vi "RFID Get ID Test-2.vi"() -> ()   [LabVIEW 2018]
uses:
  <vilib>/Instr/_visa.llb/VISA Configure Serial Port (Instr).vi
panel:
  out "error out":errorcluster
  in  "Cancel Button":bool
  in  "Get RFID":bool
  out "received":string
  in  "ComPort":refnum<visa-resource-name>="COM10"
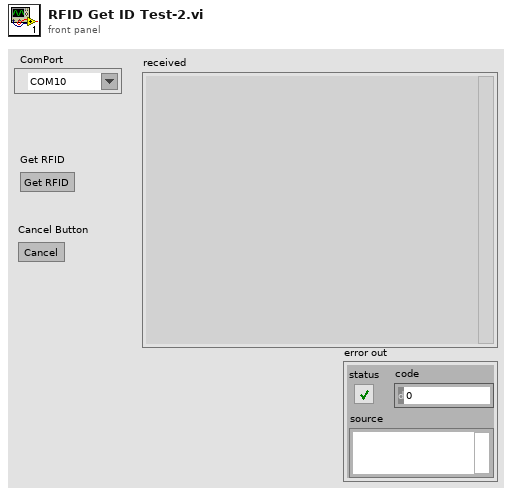
[diagram p1: front panel]
types:
  T1 = enum8{"Enabled", "Disabled", "Disabled and Grayed Out"}
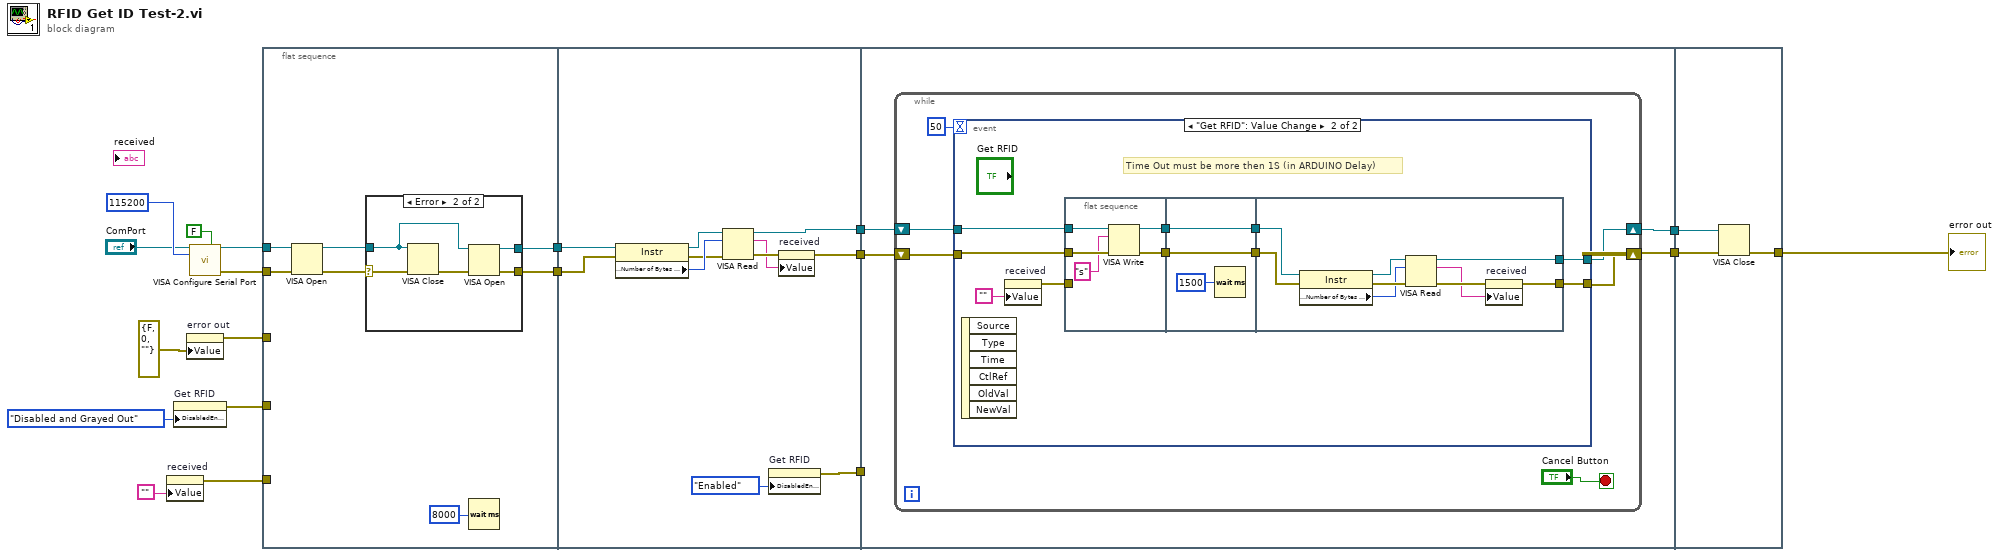
[diagram p0: block diagram]
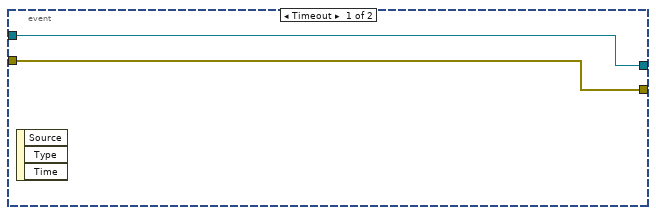
[diagram p3: hidden frame]
diagram:
  n1 = property on="received" class="Str"("Value"="") -> (error out=w13:errorcluster)  [unwired: 2 in, 1 out]
  n2 = property on="Get RFID" class="Bool"("DisabledEnum"=T1."Disabled and Grayed Out" ("Disabled")) -> (error out=w7:errorcluster)  [unwired: 2 in, 1 out]
  n3 = property on="error out" class="Clust (strict)"("Value"=errorcluster {"status"=FALSE, "code"=0, "source"=""} ("error out")) -> (error out=w1:errorcluster)  [unwired: 2 in, 1 out]
  n4 = call-poly "VISA Configure Serial Port"("VISA resource name"="ComPort", "Enable Termination\nChar (T)"=FALSE ("Enable Termination\nChar (T)"), "baud rate (9600)"=u32 115200 ("Serial Settings:Baud Rate")) -> ("VISA resource name out"=w15:refnum<visa-resource-name>, "error out"=w16:errorcluster)  [unwired: 11 in]
  n5 = flat-sequence {
    tunnel: w16 -> [w25]
    tunnel: w15 -> [w24]
    tunnel: w13 -> [_]
    tunnel: w7 -> [_]
    tunnel: [w21] -> w5
    tunnel: [w20] -> w3
    tunnel: w1 -> [_]
    tunnel: [w41] -> w14
    tunnel: [w35] -> w11
    tunnel: [w40] -> w6
    tunnel: w5 -> [w38]
    tunnel: w3 -> [w37]
    tunnel: w14 -> [w48]
    tunnel: w11 -> [w47]
    tunnel: [w46] -> w10
    tunnel: [w45] -> w9
    tunnel: w6 -> [_]
    tunnel: w10 -> [w86]
    tunnel: w9 -> [w85]
    tunnel: [w84] -> w4
    frame #0 {
      n6 = VISA Open(error in (no error)=w25, VISA resource name=w24) -> (VISA resource name=w22:refnum<visa-resource-name>, error out=w23:errorcluster)  [unwired: 3 in]
      n7 = case shown="Error" w23 {
        selector: w23 -> [w27 w33]
        tunnel: w22 -> [w28 w31]
        tunnel: [w28 w30] -> w21
        tunnel: [w27 w29] -> w20
        frame No Error {
        }
        frame Error {
          n8 = VISA Close(VISA resource name=w31, error in (no error)=w33) -> (error out=w32:errorcluster)
          n9 = VISA Open(error in (no error)=w32, VISA resource name=w31) -> (VISA resource name=w30:refnum<visa-resource-name>, error out=w29:errorcluster)  [unwired: 3 in]
        }
      }
      n10 = Wait (ms)(milliseconds to wait=u32 8000) -> ()  [unwired: 1 out]
    }
    frame #1 {
      n11 = property class="Instr"(reference=w38, error in=w37) -> (reference out=w43:refnum<visa-resource-name>, error out=w42:errorcluster, "Serial Settings:Number of Bytes at Serial Port"=w44:u32)
      n12 = VISA Read(VISA resource name=w43, byte count=w44, error in (no error)=w42) -> (VISA resource name out=w41:refnum<visa-resource-name>, read buffer=w34:string, error out=w36:errorcluster)  [unwired: 1 out]
      n13 = property on="Get RFID" class="Bool"("DisabledEnum"=T1."Enabled" ("Disabled")) -> (error out=w40:errorcluster)  [unwired: 2 in, 1 out]
      n14 = property on="received" class="Str"(error in=w36, "Value"=w34) -> (error out=w35:errorcluster)  [unwired: 1 in, 1 out]
    }
    frame #2 {
      n15 = while {
        shift-right: [w52] -> w46
        shift-left: w48 -> [w54]
        shift-right: [w51] -> w45
        shift-left: w47 -> [w53]
        stop <- "Cancel Button" stop-if-true
        n16 = event shown="[1] \"Get RFID\": Value Change" {
          selector: _ -> [_ _]
          dyn-events: _ -> [_ _]
          timeout: 50 -> [_ _]
          tunnel: w54 -> [w56 w66]
          tunnel: w53 -> [w55 w65]
          tunnel: [w56 w60] -> w52
          tunnel: [w55 w59] -> w51
          event Timeout {
            n17 = event-data() -> ()  [unwired: 1 in, 3 out]
          }
          event "Get RFID": Value Change {
            # "Time Out must be more then 1S (in ARDUINO Delay)"
            n18 = event-data() -> ()  [unwired: 1 in, 6 out]
            n19 = property on="received" class="Str"("Value"="") -> (error out=w57:errorcluster)  [unwired: 2 in, 1 out]
            n20 = flat-sequence {
              tunnel: w66 -> [w71]
              tunnel: w65 -> [w70]
              tunnel: [w68] -> w64
              tunnel: [w67] -> w63
              tunnel: w57 -> [_]
              tunnel: w64 -> [w73]
              tunnel: w63 -> [w72]
              tunnel: [w73] -> w62
              tunnel: [w72] -> w61
              tunnel: w62 -> [w80]
              tunnel: w61 -> [w79]
              tunnel: [w78] -> w60
              tunnel: [w77] -> w59
              frame #0 {
                n21 = VISA Write(VISA resource name=w71, write buffer="s", error in (no error)=w70) -> (VISA resource name out=w68:refnum<visa-resource-name>, error out=w67:errorcluster)  [unwired: 1 out]
              }
              frame #1 {
                n22 = Wait (ms)(milliseconds to wait=u32 1500) -> ()  [unwired: 1 out]
              }
              frame #2 {
                n23 = property class="Instr"(reference=w80, error in=w79) -> (reference out=w82:refnum<visa-resource-name>, error out=w83:errorcluster, "Serial Settings:Number of Bytes at Serial Port"=w81:u32)
                n24 = VISA Read(VISA resource name=w82, byte count=w81, error in (no error)=w83) -> (VISA resource name out=w78:refnum<visa-resource-name>, read buffer=w75:string, error out=w76:errorcluster)  [unwired: 1 out]
                n25 = property on="received" class="Str"(error in=w76, "Value"=w75) -> (error out=w77:errorcluster)  [unwired: 1 in, 1 out]
              }
            }
          }
        }
      }
    }
    frame #3 {
      n26 = VISA Close(VISA resource name=w86, error in (no error)=w85) -> (error out=w84:errorcluster)
    }
  }
  "error out" <- w4
